vi "Data Encapsulation.vi"() -> ()   [LabVIEW 2023]
doc: "This example demonstrates data encapsulation using LabVIEW object-oriented programming."
uses:
  Sample class/Sample Class.lvclass
  Sample class/Sample Class.lvclass/Sample Class.ctl
panel:
  out "Resulting String":string
  in  "Number":dbl
  # "Overview: Demonstrates data encapsulation with LabVIEW classes.\nInstructions:\n1. Enter a number.\n2. Run the VI.\n3. Open the block diagram and refer to the comments there."
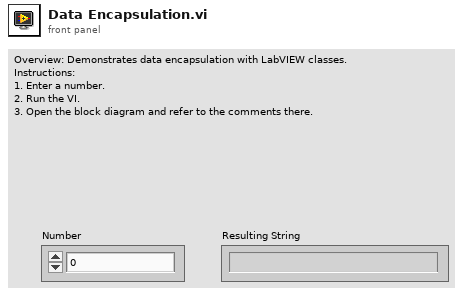
[diagram p1: front panel]
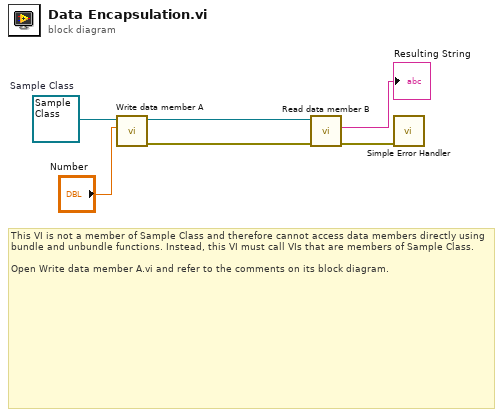
[diagram p0: block diagram]
diagram:
  w6 = refnum<class "Sample Class.lvclass"> refnum  # Sample Class
  # "This VI is not a member of Sample Class and therefore cannot access data members directly using bundle and unbundle functions. Instead, this VI must call VIs that are members of Sample Class.\n\nOpen Write data member A.vi and refer to the comments on its block diagram."
  n1 = call "Write data member A.vi"("Data member A"="Number", "Sample Class in"=w6) -> ("error out"=w2:errorcluster, "Sample Class out"=w4:refnum<class "Sample Class.lvclass">)  [unwired: 8 in]
  n2 = call "Read data member B.vi"("error in (no error)"=w2, "Sample Class in"=w4) -> ("error out"=w1:errorcluster, "data member B"=→"Resulting String":string)  [unwired: 7 in, 1 out]
  n3 = call <vilib>:"Simple Error Handler.vi"("error in (no error)"=w1) -> ()  [unwired: 4 in, 5 out]
